vi "HFRR ADV v029 new software.vi"() -> ()   [LabVIEW 2025] (continued)
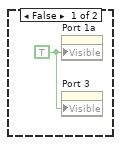
[diagram p5: hidden frame]
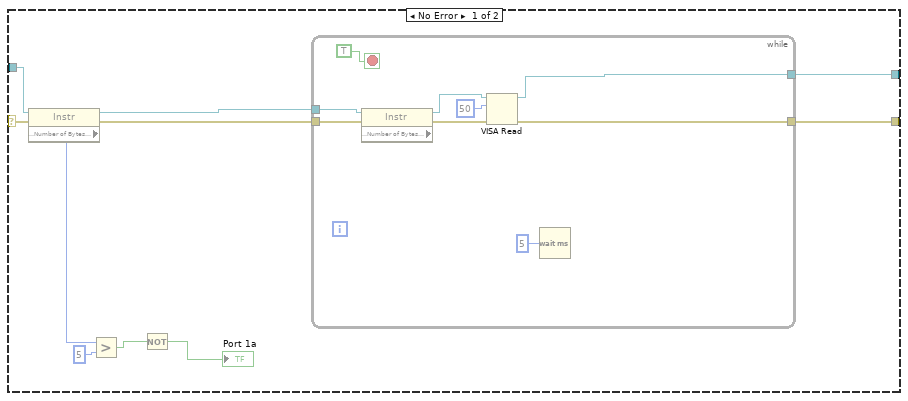
[diagram p6: hidden frame]
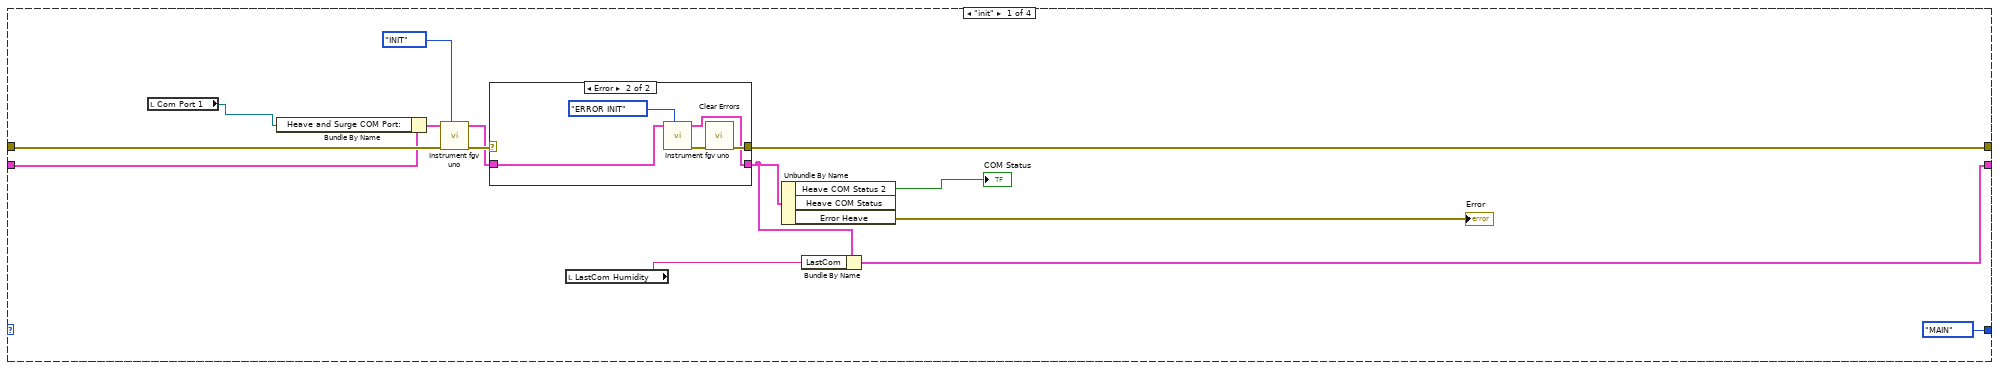
[diagram p8: hidden frame]
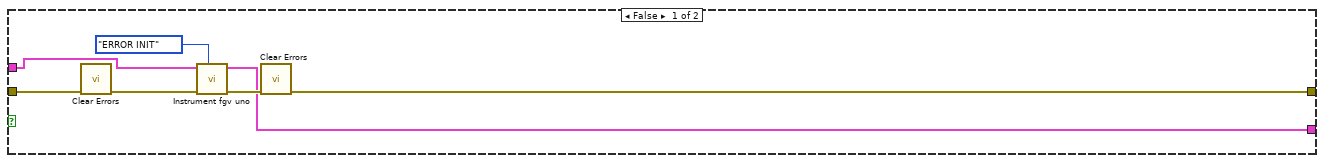
[diagram p10: hidden frame]
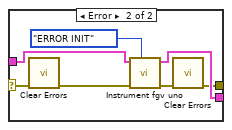
[diagram p12: hidden frame]
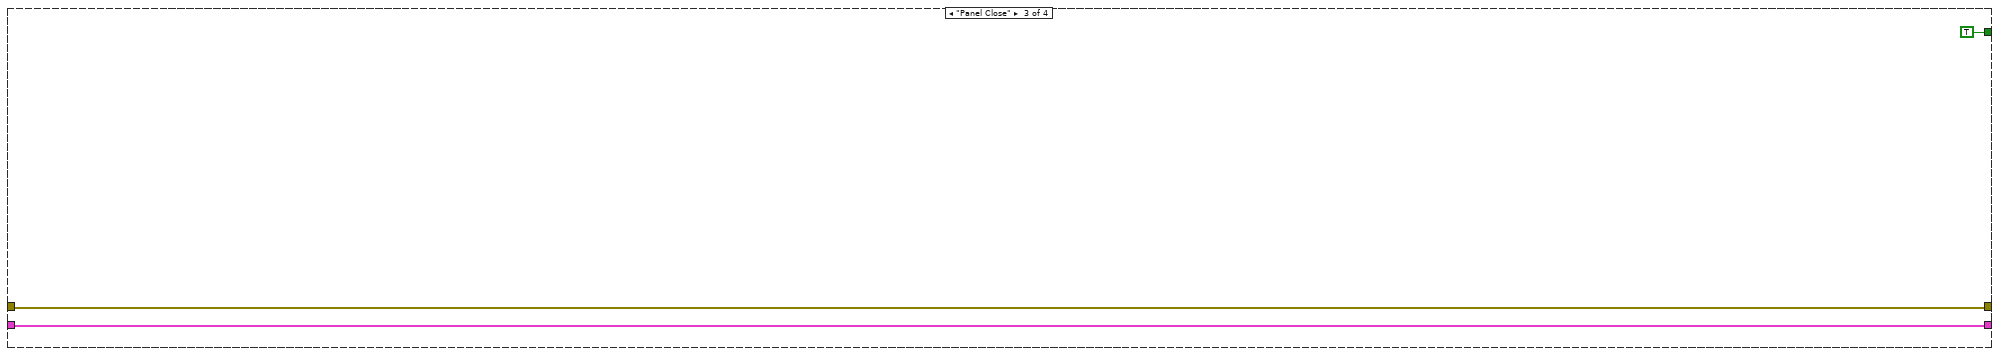
[diagram p14: hidden frame]
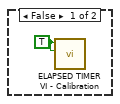
[diagram p18: hidden frame]
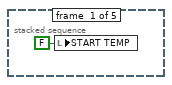
[diagram p20: hidden frame]
      }
      frame "MAIN" {
        n3362 = Unbundle By Name(w4423) -> ("Com Port 2"=w4431:refnum<visa-resource-name>)
        n3363 = local write "Com Port 4"(w4431) -> ()
        n3364 = local read "C3 :"() -> (w4421:refnum<visa-resource-name>)
        n3365 = Bundle By Name(cluster=w4423, "Heave and Surge COM Port:"=w4421) -> (w4422:T18)
        n3366 = Equal?(x=w4431, y=w4421) -> (x = y?=w4430:bool)
        n3367 = case shown="True" w4430 {
          tunnel: [w4435 w4452] -> w4429
          tunnel: w4424 -> [w4436 w4458]
          tunnel: w4422 -> [w4434 w4456]
          tunnel: [w4433 w4451] -> w4427
          frame False {
            n3368 = call <vilib>:"Clear Errors.vi"("error in (no error)"=w4436) -> ("error out"=w4432:errorcluster)  [unwired: 5 in, 1 out]
            n3369 = call "Instrument fgv.vi"("Enum"=T30."ERROR INIT", "error in (no error) 2"=w4432, "INPUT"=w4434) -> ("error"=w4438:errorcluster, "output"=w4433:T18)  [unwired: 6 in, 1 out]
            n3370 = call <vilib>:"Clear Errors.vi"("error in (no error)"=w4438) -> ("error out"=w4435:errorcluster)  [unwired: 5 in, 1 out]
          }
          frame True {
            n3371 = call "Instrument fgv.vi"("Enum"=T30."READ", "error in (no error) 2"=w4458, "INPUT"=w4456) -> ("error"=w4457:errorcluster, "output"=w4449:T18)  [unwired: 6 in, 1 out]
            n3372 = Bundle By Name(cluster=w4449, "String 36"="WRITE UNO") -> (w4448:T18)
            n3373 = case shown="True" "Write S" {
              selector: "Write S" -> [_ w4478]
              tunnel: w4457 -> [w4471 w4477]
              tunnel: [w4471 w4476] -> w4446
              tunnel: w4448 -> [w4470 w4473]
              tunnel: [w4470 w4472] -> w4445
              frame False {
              }
              frame True {
                n3374 = Not(x=w4478) -> (.not. x?=w4474:bool)
                n3375 = local write "Write S"(w4474) -> ()
                n3376 = call "Instrument fgv.vi"("Enum"=T30."MANUAL WRITE", "error in (no error) 2"=w4477, "INPUT"=w4473) -> ("error"=w4476:errorcluster, "output"=w4472:T18)  [unwired: 6 in, 1 out]
              }
            }
            n3377 = Array Size(array="Write UNO") -> (size(s)=w4443:i32)
            n3378 = Greater Than 0?(x=w4443) -> (x > 0?=w4442:bool)
            n3379 = call "Instrument fgv.vi"("Enum"=T30."WRITE", "error in (no error) 2"=w4446, "WriteCC1"="Write UNO", "INPUT"=w4445) -> ("error"=w4454:errorcluster, "WriteCC1 2"=w4444:string[], "output"=w4453:T18)  [unwired: 5 in]
            n3380 = case shown="True" w4442 {
              tunnel: w4444 -> [_ w4460]
              frame False {
              }
              frame True {
                n3381 = local write "Write UNO"(w4460) -> ()
              }
            }
            n3382 = case shown="Error" w4454 {
              selector: w4454 -> [w4461 w4464]
              tunnel: w4453 -> [w4462 w4469]
              tunnel: [w4462 w4468] -> w4451
              tunnel: [w4461 w4466] -> w4452
              frame No Error {
              }
              frame Error {
                n3383 = call <vilib>:"Clear Errors.vi"("error in (no error)"=w4464) -> ("error out"=w4463:errorcluster)  [unwired: 5 in, 1 out]
                n3384 = call "Instrument fgv.vi"("Enum"=T30."ERROR INIT", "error in (no error) 2"=w4463, "INPUT"=w4469) -> ("error"=w4467:errorcluster, "output"=w4468:T18)  [unwired: 6 in, 1 out]
                n3385 = call <vilib>:"Clear Errors.vi"("error in (no error)"=w4467) -> ("error out"=w4466:errorcluster)  [unwired: 5 in, 1 out]
              }
            }
            n3386 = Unbundle By Name(w4451) -> ("LastCom"=→"LastCom UNO":string, "Read Heave and Surge"=→"Read UNO":string)
          }
        }
        n3387 = Unbundle By Name(w4427) -> ("Heave COM Status 2"=w4428:bool, "Heave COM Status"=w4416:bool, "Error Heave"=w4414:errorcluster, "Bytes at Heave Port"=→"Bytes at Humidity Port":dbl)
        n3388 = Unbundle By Name(w4414) -> ()  [unwired: 1 out]
        n3389 = Not(x=w4416) -> (.not. x?=w4425:bool)
        n3390 = Not(x=w4428) -> (.not. x?=w4415:bool)
        n3391 = local write "Instrument Status"(w4425) -> ()
        n3392 = local write "Error  2"(w4414) -> ()
        n3393 = local write "Port 1a"(w4416) -> ()
        n3394 = local read "Quit"() -> (w4418:bool)
        n3395 = local write "COM Status"(w4415) -> ()
        n3396 = Select(t=enum16{"init", "MAIN", "Panel Close"}."Panel Close", s=w4418, f=enum16{"init", "MAIN", "Panel Close"}."MAIN") -> (s? t:f=w4417:enum16{"init", "MAIN", "Panel Close"})
      }
      frame "Panel Close" {
      }
      frame Default {
      }
    }
  }
  n3397 = while {
    stop <- w4509 stop-if-true
    n3398 = local read "Read HUMIDITY"() -> (w4484:string)
    n3399 = call <vilib>:"High Resolution Polling Wait.vi"("seconds to wait"=0.05) -> ()  [unwired: 10 in, 1 out]
    n3400 = Spreadsheet String To Array(delimiter (Tab)=",", format string="", spreadsheet string=w4484, array type (2D Dbl)=string[] []) -> (array=w4504:string[])
    n3401 = for {
      tunnel: w4504 -> [w4514] mode=indexing
      tunnel: string[] ["STATE;", "SET;", "RH;", "T;", "AMB_RH;", "AMB_T;", "PUMP;", "FAN_IN;", "FAN_OUT;", "DEHUM;", "CURRENT;", "STALL;"] -> [w4513] mode=indexing
      tunnel: [w4512] -> w4503 mode=indexing
      n3402 = Match Pattern(string=w4514, regular expression=w4513) -> (after substring=w4512:string)  [unwired: 1 in, 3 out]
    }
    n3403 = Index Array(array=w4503) -> (element #1=→"STATE :":string, element #2=→"SET :":string, element #3=w4492:string, element #4=→"T :":string, element #5=w4490:string, element #6=→"AMB_T :":string, element #7=→"PUMP :":string, element #8=→"FAN_IN :":string, element #9=→"FAN_OUT :":string, element #10=→"DEHUM :":string, element #11=→"CURRENT :":string, element #12=→"STALL :":string)  [unwired: 12 in]
    "RH :" <- w4492
    "AMB_RH :" <- w4490
    n3404 = Fract/Exp String To Number(string=w4492) -> (number=w4485:dbl)  [unwired: 3 in, 1 out]
    n3405 = Fract/Exp String To Number(string=w4490) -> (number=w4489:dbl)  [unwired: 3 in, 1 out]
    n3406 = local write "Ambient Humidity :"(w4489) -> ()
    n3407 = Equal?(x=w4485, y=0.0) -> (x = y?=w4487:bool)
    n3408 = case shown="True" w4487 {
      tunnel: [w4510 w4511] -> w4486
      tunnel: w4485 -> [w4510 _]
      frame False {
        (unwired) 0.0
        "Humidity temp" <- w4510
      }
      frame True {
        n3409 = local read "Humidity temp"() -> (w4511:dbl)
      }
    }
    "RH Numeric:" <- w4486
    n3410 = local read "Quit"() -> (w4509:bool)
  }
